vi "Create Client.vi"(8 "error in (no error)":errorcluster, 10 "certificatePath":string, 11 "address":string) -> (0 "error out":errorcluster, 3 "gRPC Client out":refnum<class "Template Client.lvclass">)   [LabVIEW 2019, in "Template Client.lvlib" / "Template Client.lvclass"]
uses:
  Template Client.lvclass
  Template Client.lvclass/Template Client.ctl
  <vilib>/gRPC/LabVIEW gRPC Library/gprc-lvsupport-release.lvlib
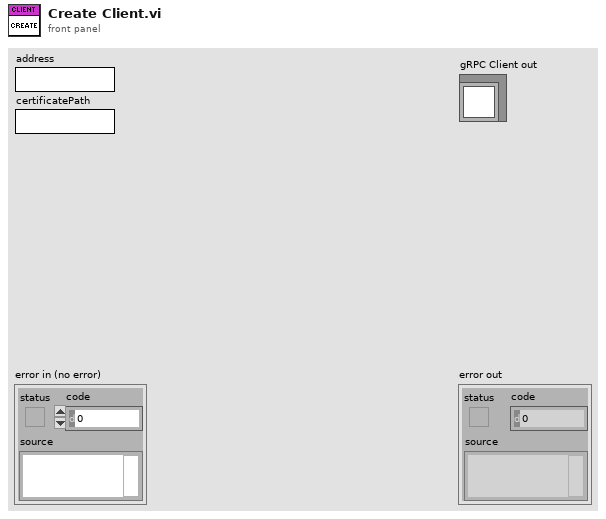
[diagram p1: front panel]
types:
  T1 = typedef "gprc-lvsupport-release.lvlib/grpcId.ctl" = u64
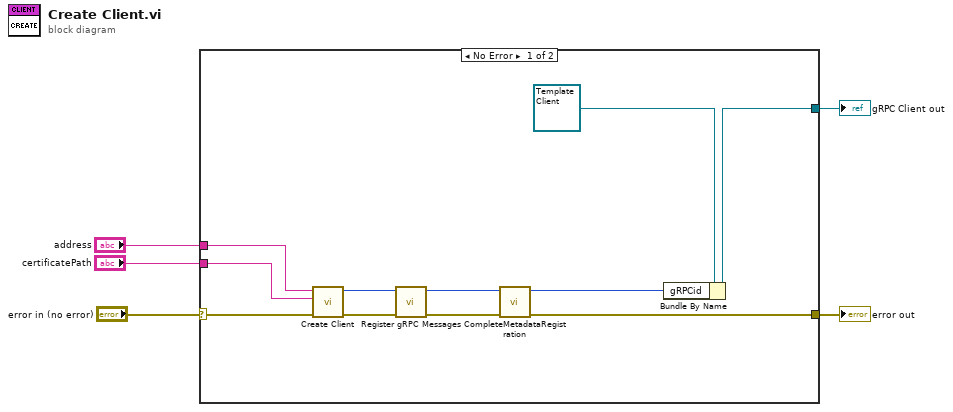
[diagram p0: block diagram]
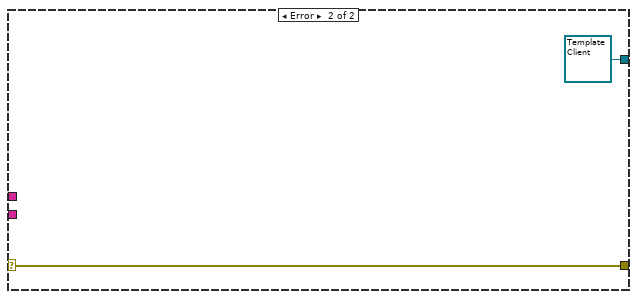
[diagram p2: hidden frame]
diagram:
  n1 = case shown="No Error" "error in (no error)" {
    selector: "error in (no error)" -> [w16 w18]
    tunnel: [w9 w18] -> w4
    tunnel: "address" -> [w15 _]
    tunnel: "certificatePath" -> [w14 _]
    tunnel: [w6 refnum<class "Template Client.lvclass"> refnum ("Template Client out")] -> w1
    frame No Error {
      n2 = call <vilib>:"Create Client.vi"("error in (no error)"=w16, "certificatePath"=w14, "address"=w15) -> ("error out"=w12:errorcluster, "Client Ref Out"=w13:T1)  [unwired: 7 in]
      n3 = call "Register gRPC Messages.vi"("error in (no error)"=w12, "gRPCid"=w13) -> ("error out"=w10:errorcluster, "gRPCid"=w11:T1)  [unwired: 8 in]
      n4 = call <vilib>:"CompleteMetadataRegistration.vi"("error in (no error)"=w10, "gRPC ID"=w11) -> ("error out"=w9:errorcluster, "gRPC ID Out"=w8:T1)  [unwired: 8 in]
      n5 = Bundle By Name(cluster=refnum<class "Template Client.lvclass"> refnum ("Template Client out"), "gRPCid"=w8) -> (w6:refnum<class "Template Client.lvclass">)
    }
    frame Error {
    }
  }
  "error out" <- w4
  "gRPC Client out" <- w1
